vi "test_Add Command.vi"(8 "error in (no error)":errorcluster, 11 "TestCase in":refnum<class "Instrument Addon Scripting API Messages Unit Tests.lvclass">) -> (0 "error out":errorcluster, 3 "TestCase out":refnum<class "Instrument Addon Scripting API Messages Unit Tests.lvclass">)   [LabVIEW 2018, in "Instrument Addon Scripting API Messages Unit Tests.lvclass"]
uses:
  Instrument Addon Scripting API Messages Unit Tests.lvclass
  <vilib>/NI Veristand/Custom Device API/Custom Device Item Ref.ctl
  Addon/Addon Shared/Types/FG Control.ctl
  APIs/Scripting API/TypeDefs/Command Settings.ctl
  APIs/Scripting API/TypeDefs/Padding.ctl
  APIs/Scripting API/TypeDefs/Linked Channel.ctl
  NationalInstruments.VeriStand.SystemDefinitionAPI
  APIs/Scripting API/TypeDefs/Message Settings.ctl
  APIs/Scripting API/TypeDefs/Protection Types.ctl
  Addon/Addon Shared/SubVIs/Constants.vi
  <vilib>/NI Veristand/Custom Device Tools/Custom Device Utility Library/NI VeriStand - Search for Item by GUID.vi
  APIs/Scripting API/Messages/Create Message - Trigger Only.vi
  <vilib>/NI Veristand/Custom Device API/NI VeriStand - Get Item Property.vi
  <vilib>/NI Veristand/Custom Device API/Get Item Property (Boolean).vi
  <vilib>/NI Veristand/Custom Device API/Get Item Property (String).vi
  <vilib>/NI Veristand/Custom Device API/NI VeriStand - Set Item Property.vi
  <vilib>/NI Veristand/Custom Device API/Set Item Property (Boolean).vi
  <vilib>/NI Veristand/Custom Device API/Set Item Property (String).vi
  <vilib>/NI Veristand/Custom Device API/Get Item Property (U32).vi
  <vilib>/NI Veristand/Custom Device API/Get Item Property (Double).vi
  <vilib>/NI Veristand/Custom Device API/Set Item Property (U32).vi
  <vilib>/NI Veristand/Custom Device API/Set Item Property (Double).vi
  <vilib>/addons/_JKI Toolkits/VI Tester/TestCase.llb/TestCase.lvclass
  Instrument Addon Scripting API Test Assets/Instrument Addon Scripting API Test Assets.lvclass
  APIs/Scripting API/Instrument Addon Scripting API.lvlib
  <vilib>/NI VeriStand/Custom Device Tools/Custom Device Utility Library/Custom Device Utility Library.lvlib
  Addon/Addon Shared/Instrument Addon Shared.lvlib
  <vilib>/NI VeriStand/Custom Device API/Custom Device API.lvlib
  C:/Program Files (x86)/National Instruments/LabVIEW 2018/vi.lib/addons/_JKI Toolkits/VI Tester/TestCase.llb/TestCase.lvclass
panel:
  out "GUID 2":string
  out "Item Ref":T1 format="%.0x"
  out "Channel Ref Out":T1 format="%.0x"
  out "GUID":string
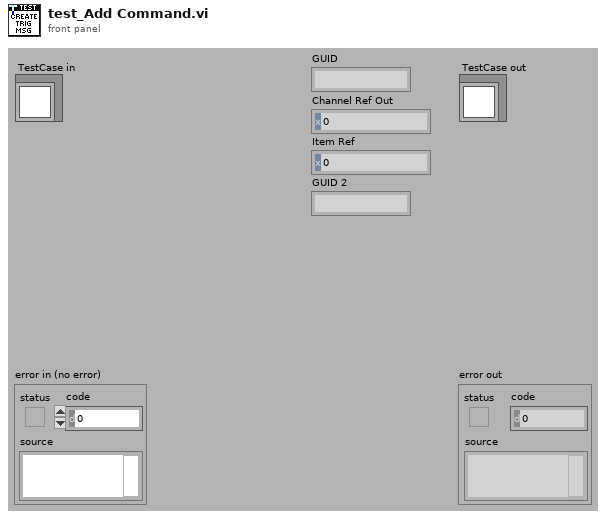
[diagram p1: front panel]
types:
  T1 = typedef "Custom Device API.lvlib/Custom Device Item Ref.ctl" = u64
  T2 = typedef "Instrument Addon Scripting API.lvlib/Command Settings.ctl" = cluster{"Command Format":string, "Use Padding?":bool, "Padding":T3, "Linkages":T4}
  T3 = typedef "Instrument Addon Scripting API.lvlib/Padding.ctl" = cluster{"Length":u32, "Pad Value":u8}
  T4 = typedef "Instrument Addon Scripting API.lvlib/Linked Channel.ctl" = cluster{"Channel Ref":T1, "Variable Name":string}[]
  T5 = typedef "Instrument Addon Shared.lvlib/FG Control.ctl" = enum16{"Get", "Set"}
  T6 = typedef "Instrument Addon Scripting API.lvlib/Message Settings.ctl" = cluster{"Protection Types":T7, "Enable Periodic Default":bool, "Trigger Channel Refnum":u64}
  T7 = typedef "Instrument Addon Scripting API.lvlib/Protection Types.ctl" = enum16{"None", "CRC-32", "Checksum U16", "Checksum U32", "Checksum U8"}
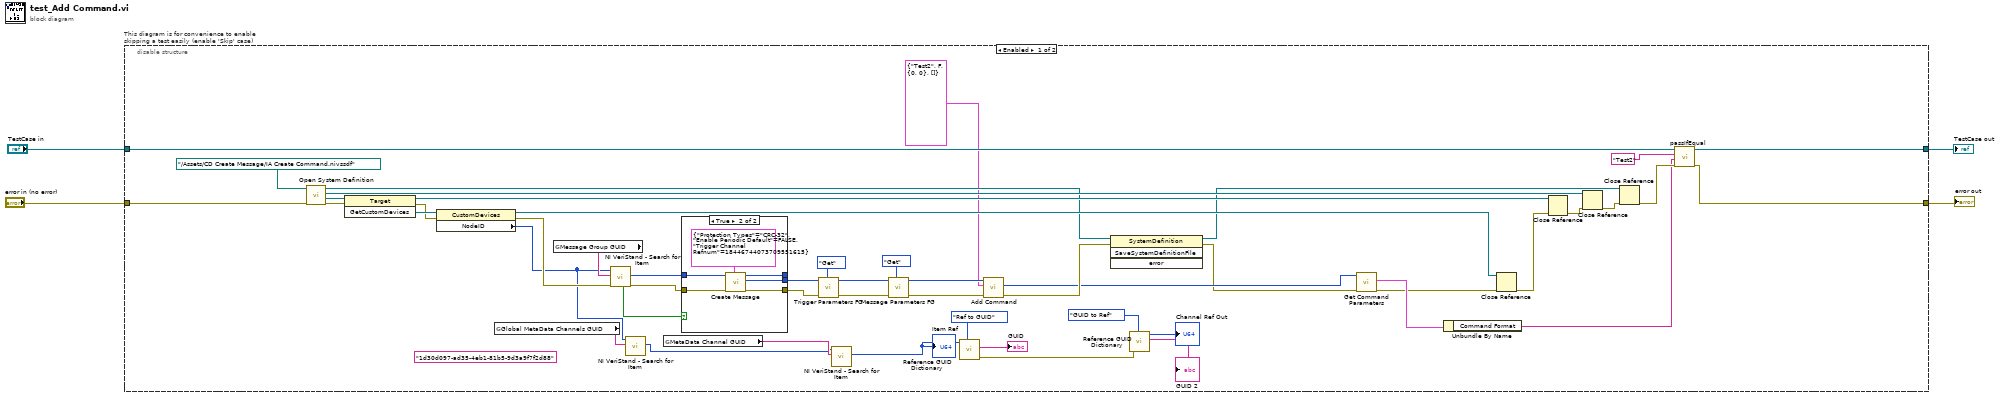
[diagram p0: block diagram]
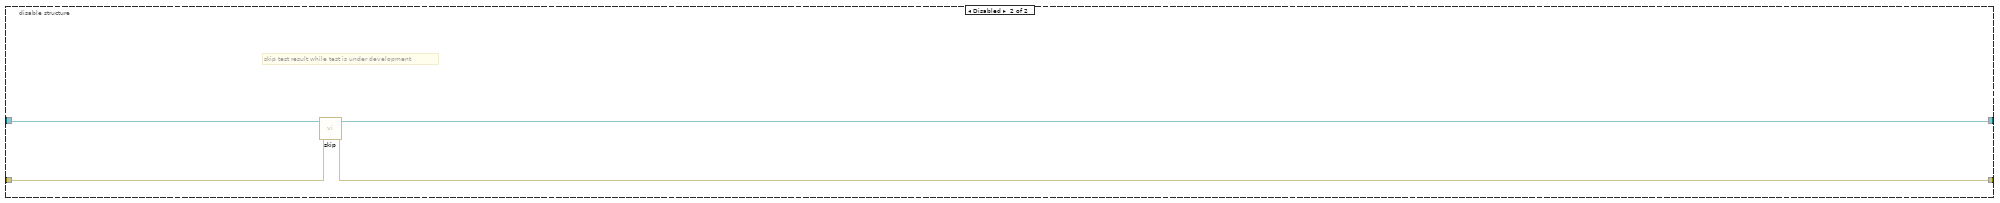
[diagram p3: hidden frame]
diagram:
  n1 = disable-structure "This diagram is for convenience to enable skipping a test easily (enable 'Skip' case)" shown="Enabled" {
    disable-tunnel: "TestCase in" -> [w36 w65]
    disable-tunnel: [w32 w63] -> w1
    disable-tunnel: [w33 w64] -> w3
    disable-tunnel: "error in (no error)" -> [w53 w62]
    frame Enabled {
      (unwired) "1d30d097-ad35-4eb1-81b5-9d3a9f7f2d88" ("MetaData Channel GUID")
      n2 = call "Open System Definition.vi"("error in (no error)"=w53, "System Definition File"=path "../Assets/CD Create Message/IA Create Command.nivssdf" ("SDF file")) -> ("error out"=w47:errorcluster, "Target Refnum"=w52:refnum<k24>, "Root Refnum"=w42:refnum<k24>, "System Definition Refnum"=w24:refnum<k24>)  [unwired: 6 in]
      n3 = invoke class="Target" method="GetCustomDevices"(reference=w52, error in=w47) -> (reference out=w30:refnum<k24>, error out=w46:errorcluster, "GetCustomDevices"=w51:refnum<k24>)  [unwired: 1 in]
      n4 = property class="CustomDevices"(reference=w51, error in=w46) -> (reference out=w43:refnum<k24>, error out=w45:errorcluster, "NodeID"=w14:u64)
      n5 = global read "Constants.vi" "Global MetaData Channels GUID"() -> (w15:string)
      n6 = global read "Constants.vi" "Message Group GUID"() -> (w50:string)
      n7 = call-poly <vilib>:"NI VeriStand - Search for Item.vi"("error in"=w45, "Item GUID"=w50, "Section Ref in"=w14) -> ("error out"=w44:errorcluster, "Item Ref"=w49:T1, "Found"=w48:bool)  [unwired: 5 in, 1 out]
      n8 = call-poly <vilib>:"NI VeriStand - Search for Item.vi"("Item GUID"=w15, "Section Ref in"=w14) -> ("Item Ref"=w12:T1)  [unwired: 6 in, 3 out]
      n9 = global read "Constants.vi" "MetaData Channel GUID"() -> (w13:string)
      n10 = case shown="True" w48 {
        tunnel: w49 -> [_ w61]
        tunnel: [w55 w60] -> w37
        tunnel: w44 -> [w55 w59]
        tunnel: [_ w58] -> w31
        tunnel: [_ w57] -> _
        frame False {
        }
        frame True {
          n11 = call-poly "Create Message.vi"("Message Settings"=T6 {"Protection Types"=enum."CRC-32", "Enable Periodic Default"=FALSE, "Trigger Channel Refnum"=18446744073709551615}, "error in (no error)"=w59, "Message Group in"=w61) -> ("error out"=w60:errorcluster, "Message Refnum out"=w58:T1, "Message Goup out"=w57:T1)  [unwired: 6 in]
        }
      }
      n12 = call "Trigger Parameters FG.vi"("Action"=FG_Control."Get", "error in (no error)"=w37, "Item Ref in"=w31) -> ("error out"=w40:errorcluster, "Item Ref out"=w41:T1)  [unwired: 6 in, 1 out]
      n13 = call-poly <vilib>:"NI VeriStand - Search for Item.vi"("Item GUID"=w13, "Section Ref in"=w12) -> ("Item Ref"=w10:T1)  [unwired: 6 in, 3 out]
      "Item Ref" <- w10
      n14 = call "Message Parameters FG.vi"("Action"=FG_Control."Get", "error in (no error)"=w40, "Item Ref in"=w41) -> ("error out"=w26:errorcluster, "Item Ref out"=w27:T1)  [unwired: 6 in, 1 out]
      n15 = call "Reference GUID Dictionary.vi"("Enum"=enum16{"Ref to GUID", "GUID to Ref"}."Ref to GUID", "Channel Ref"=w10) -> ("error out"=w7:errorcluster, "GUID"=→"GUID":string)  [unwired: 7 in, 1 out]
      n16 = call "Add Command.vi"("error in (no error)"=w26, "Settings"=T2 {"Command Format"="Test2", "Use Padding?"=FALSE, "Padding"={"Length"=0, "Pad Value"=0}, "Linkages"=[]}, "Message Refnum In"=w27) -> ("error out"=w25:errorcluster, "Command Refnum"=w20:T1)  [unwired: 6 in, 1 out]
      n17 = invoke class="SystemDefinition" method="SaveSystemDefinitionFile"(reference=w24, error in=w25) -> (reference out=w23:refnum<k24>, error out=w19:errorcluster)  [unwired: 2 in, 2 out]
      n18 = call "Reference GUID Dictionary.vi"("Enum"=enum16{"Ref to GUID", "GUID to Ref"}."GUID to Ref", "error in"=w7) -> ("GUID"=→"GUID 2":string, "Channel Ref Out"=→"Channel Ref Out":T1)  [unwired: 7 in, 1 out]
      n19 = call "Get Command Parameters.vi"("error in (no error)"=w19, "Item Ref in"=w20) -> ("error out"=w17:errorcluster, "Command Parameters Out"=w18:T2)  [unwired: 7 in, 1 out]
      n20 = Unbundle By Name(w18) -> ("Command Format"=w22:string)
      n21 = Close Reference(reference=w43, error in (no error)=w17) -> (error out=w29:errorcluster)
      n22 = Close Reference(reference=w30, error in (no error)=w29) -> (error out=w28:errorcluster)
      n23 = Close Reference(reference=w42, error in (no error)=w28) -> (error out=w35:errorcluster)
      n24 = Close Reference(reference=w23, error in (no error)=w35) -> (error out=w34:errorcluster)
      n25 = call-dynamic "passIfEqual.vi"("error in (no error)"=w34, "y"=w22, "x"="Test2" ("Command"), "TestCase in"=w36) -> ("error out"=w33:errorcluster, "TestCase out"=w32:refnum<class "Instrument Addon Scripting API Messages Unit Tests.lvclass">)  [unwired: 6 in]
    }
    frame Disabled {
      # "skip test result while test is under development"
      n26 = call <vilib>:"skip.vi"("error in (no error)"=w62, "TestCase in"=w65) -> ("error out"=w64:errorcluster, "TestCase out"=w63:refnum<class "Instrument Addon Scripting API Messages Unit Tests.lvclass">)  [unwired: 8 in]
    }
  }
  "error out" <- w3
  "TestCase out" <- w1
